vi "Convert_Lat-Long_to_UTM.vi"() -> ()   [LabVIEW 2011]
panel:
  out "X":dbl format="%.4f"
  out "Y":dbl format="%.4f"
  in  "NH (Spindle Number)":dbl format="%.2f"
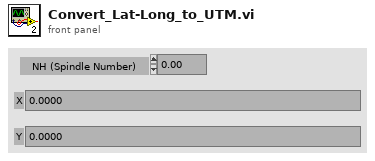
[diagram p1: front panel]
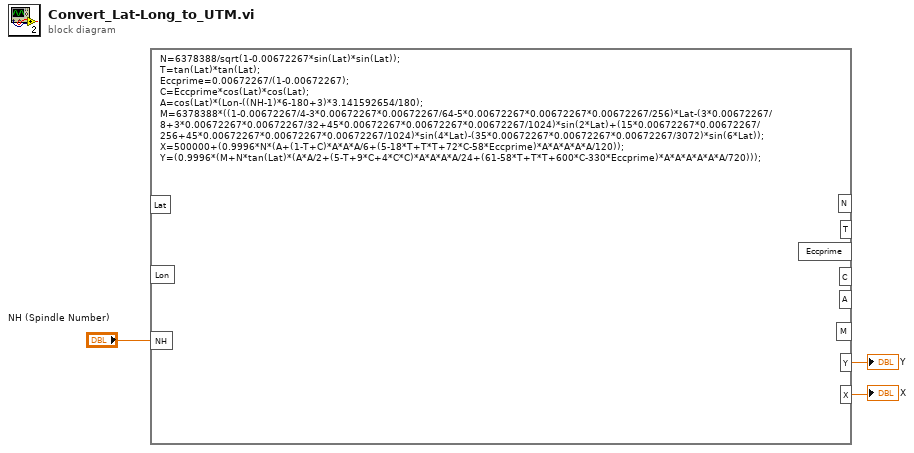
[diagram p0: block diagram]
diagram:
  n1 = formula code="N=6378388/sqrt(1-0.00672267*sin(Lat)*sin(Lat));\nT=tan(Lat)*tan(Lat);\nEccprime=0.00672267/(1-0.00672267);\nC=Eccprime*cos(Lat)*cos(Lat);\nA=cos(Lat)*(Lon-((NH-1)*6-180+3)*3.141592654/180);\nM=6378388*((1-0.00672267/4-3*0.00672267*0.00672267/64-5*0.00672267*0.00672267*0.00672267/256)*Lat-(3*0.00672267/8+3*0.00672267*0.00672267/32+45*0.00672267*0.00672267*0.00672267/1024)*sin(2*Lat)+(15*0.00672267*0.00672267/256+45*0.00672267*0.00672267*0.00672267/1024)*sin(4*Lat)-(35*0.00672267*0.00672267*0.00672267/3072)*sin(6*Lat));\nX=500000+(0.9996*N*(A+(1-T+C)*A*A*A/6+(5-18*T+T*T+72*C-58*Eccprime)*A*A*A*A*A/120));\nY=(0.9996*(M+N*tan(Lat)*(A*A/2+(5-T+9*C+4*C*C)*A*A*A*A/24+(61-58*T+T*T+600*C-330*Eccprime)*A*A*A*A*A*A/720)));"("NH"="NH (Spindle Number)") -> ("Y"=→"Y":dbl, "X"=→"X":dbl)  [unwired: 2 in, 6 out]
